vi "Is Support Trigger Sense.vi"() -> (3 "function return":i32)   [LabVIEW 2021, in "vmmso.lvlib"]
doc: "DLL_API int WINAPI IsSupportTriggerSense();"
uses:
  vmmso.lvlib
  vmmso.dll
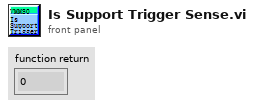
[diagram p1: front panel]
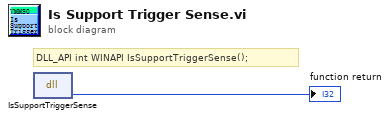
[diagram p0: block diagram]
diagram:
  # "DLL_API int WINAPI IsSupportTriggerSense();"
  n1 = dll-call lib="D:/labviewdemo/LabviewDemo 21/vmmso/vmmso.*" fn="IsSupportTriggerSense"() -> (→"function return":i32)  [unwired: 3 in, 2 out]
